vi "OpenReport.vi"(8 "error in (no error)":errorcluster) -> (0 "error out":errorcluster)   [LabVIEW 2018, in "File IO.lvlib"]
doc: "This subVI enqueues the named action in to the communications queue along with the input data."
uses:
  File IO.lvlib
  Private Controls/Module Data.ctl
  Private Controls/Module Action.ctl
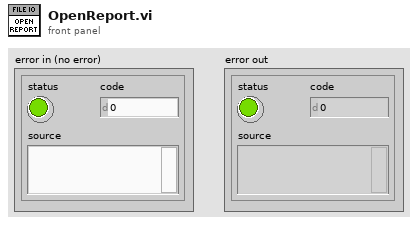
[diagram p1: front panel]
types:
  T1 = typedef "File IO.lvlib/Module Data.ctl" = cluster{"Data":variant, "Action":T2}
  T2 = typedef "File IO.lvlib/Module Action.ctl" = enum8{"Timeout", "OpenReport", "Continue Test", "Init", "Error", "Exit", "Save Accel Data", "Set Recording State", "Start New Test", "Write to System Log", "Save Stored APU Data", "Load APU Setup File", "Increment Run Count", "Write To Report"}
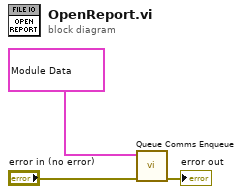
[diagram p0: block diagram]
diagram:
  n1 = call "Queue Comms Enqueue.vi"("error in (no error)"="error in (no error)", "element"=T1 {"Data"=variant, "Action"=enum."OpenReport"}) -> ("error out"=→"error out":errorcluster)  [unwired: 9 in]
